vi "initPort.vi"(5 "VISA resource name":refnum<visa-resource-name>) -> (0 "error out":errorcluster, 2 "reference out":refnum<visa-resource-name>)   [LabVIEW 2010]
uses:
  <vilib>/Instr/_visa.llb/VISA Configure Serial Port (Instr).vi
panel:
  in  "flow control":u16(ring) caption="流程控制" items=["无"=0, "XON/XOFF"=1, "RTS/CTS"=2, "DTR/DSR"=4]
  in  "End write with termination character?":bool=TRUE caption="终止符时结束写入？"
  in  "Input\nbuffer size":u32=4096 caption="输入缓冲区大小"
  in  "XOFF Character":u8=19 caption="XOFF字符" format="%.0x"
  in  "XON Character":u8=17 caption="XON字符" format="%.0x"
  in  "termination char\n(0xA = '\\n' = LF)":u8=22 caption="终止符\n(0xA = '\\n' = LF)" format="%.0x"
  in  "End read on termination character?":bool=TRUE caption="终止符时结束读取？"
  in  "timeout (ms)":u32=500 caption="超时(ms)"
  in  "parity":u16(ring)=2 caption="奇偶校验" items=["无", "奇", "偶", "标记", "空格"]
  in  "data bits":u16=8 caption="数据比特" min=5 max=8 step=1
  in  "stop bits":u16(ring)=10 caption="停止位" items=["1.0"=10, "1.5"=15, "2.0"=20]
  in  "baud rate":u32=2400 caption="波特率"
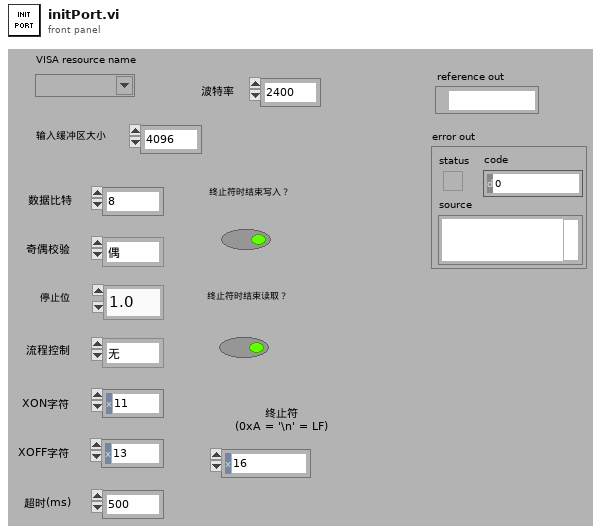
[diagram p1: front panel]
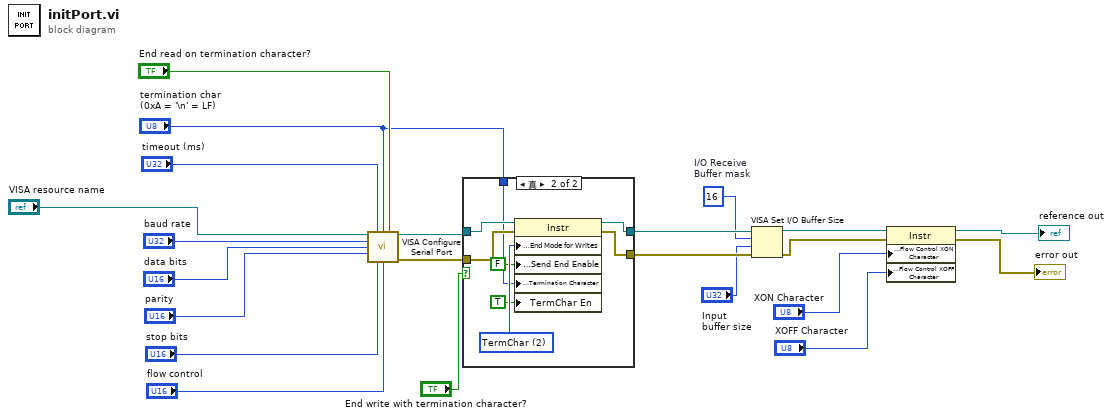
[diagram p0: block diagram]
diagram:
  w10 = u16 16  # I/O Receive Buffer mask
  n1 = call-poly "VISA Configure Serial Port"("VISA resource name"="VISA resource name", "timeout (10sec)"="timeout (ms)", "termination char\n(0xA = '\\n' = LF)"="termination char\n(0xA = '\\n' = LF)", "Enable Termination\nChar (T)"="End read on termination character?", "baud rate (9600)"="baud rate", "data bits (8)"="data bits", "parity (0:none)"="parity", "stop bits (10: 1 bit)"="stop bits", "flow control (0:none)"="flow control") -> ("VISA resource name out"=w15:refnum<visa-resource-name>, "error out"=w13:errorcluster)  [unwired: 1 in, 4 out]
  n2 = case shown="真" "End write with termination character?" {
    tunnel: w15 -> [w24 w32]
    tunnel: w13 -> [w23 w31]
    tunnel: [w24 w29] -> w12
    tunnel: [w23 w28] -> w11
    tunnel: "termination char\n(0xA = '\\n' = LF)" -> [_ w27]
    frame False {
    }
    frame True {
      w30 = u16 2 items=["None", "LastBit", "TermChar", "Break"] ("Serial Settings:Serial End Mode for Writes")
      n3 = property class="Instr"(reference=w32, error in=w31, "Serial Settings:End Mode for Writes"=w30, "Message Based Settings:Send End Enable"=FALSE, "Message Based Settings:Termination Character"=w27, "TermChar En"=TRUE ("Message Based Settings:Termination Character Enable")) -> (reference out=w29:refnum<visa-resource-name>, error out=w28:errorcluster)
    }
  }
  n4 = VISA Set I/O Buffer Size(VISA resource name=w12, mask (16)=w10, size (4096)="Input\nbuffer size", error in (no error)=w11) -> (VISA resource name out=w8:refnum<visa-resource-name>, error out=w7:errorcluster)
  n5 = property class="Instr"(reference=w8, error in=w7, "Serial Settings:Flow Control XON Character"="XON Character", "Serial Settings:Flow Control XOFF Character"="XOFF Character") -> (reference out=→"reference out":refnum<visa-resource-name>, error out=→"error out":errorcluster)
